vi "spill_param_tcp_server_v2.vi"(6 "error in":errorcluster, 8 "spill_id_Refnum":refnum<vi>, 9 "EOS_Refnum":refnum<vi>, 10 "BOS_Refnum":refnum<vi>, 11 "port":i16=9999) -> (4 "error out":errorcluster)   [LabVIEW 2019]
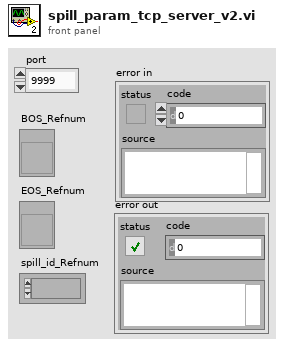
[diagram p1: front panel]
types:
  T1 = enum16{"Standard", "Buffered", "CRLF", "Immediate"}
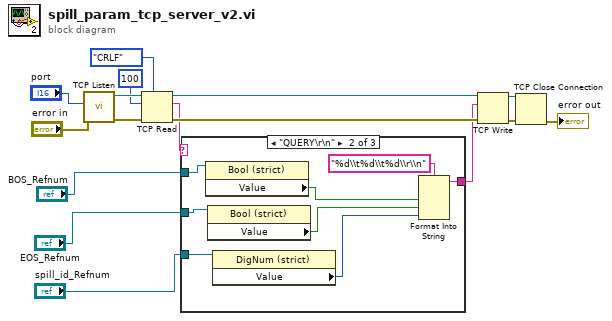
[diagram p0: block diagram]
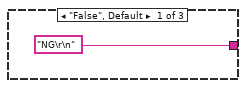
[diagram p2: hidden frame]
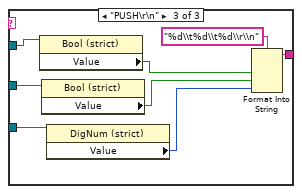
[diagram p3: hidden frame]
diagram:
  n1 = call <vilib>:"TCP Listen.vi"("error in (no error)"="error in", "port"="port") -> ("error out"=w16:errorcluster, "connection ID"=w15:refnum<k5>)  [unwired: 5 in, 3 out]
  n2 = TCP Read(connection ID=w15, bytes to read=100, error in (no error)=w16, 7:T1."CRLF" ("mode (standard)")) -> (connection ID out=w13:refnum<k5>, data out=w6:string, error out=w14:errorcluster)  [unwired: 1 in]
  n3 = case shown="\"QUERY\\r\\n\"" w6 {
    tunnel: ["NG\r\n" w24 w32] -> w9
    tunnel: "BOS_Refnum" -> [_ w23 w31]
    tunnel: "EOS_Refnum" -> [_ w21 w30]
    tunnel: "spill_id_Refnum" -> [_ w19 w29]
    frame "False", Default {
    }
    frame "QUERY\r\n" {
      n4 = property on="Property Node" class="Bool (strict)"(reference=w23) -> ("Value"=w22:bool)  [unwired: 1 in, 2 out]
      n5 = property on="Property Node" class="Bool (strict)"(reference=w21) -> ("Value"=w20:bool)  [unwired: 1 in, 2 out]
      n6 = property on="Property Node" class="DigNum (strict)"(reference=w19) -> ("Value"=w18:i32)  [unwired: 1 in, 2 out]
      n7 = Format Into String(format string="%d\\t%d\\t%d\\r\\n", w22, w20, w18) -> (resulting string=w24:string)  [unwired: 2 in, 1 out]
    }
    frame "PUSH\r\n" {
      n8 = property on="Property Node" class="Bool (strict)"(reference=w31) -> ("Value"=w28:bool)  [unwired: 1 in, 2 out]
      n9 = property on="Property Node" class="Bool (strict)"(reference=w30) -> ("Value"=w27:bool)  [unwired: 1 in, 2 out]
      n10 = property on="Property Node" class="DigNum (strict)"(reference=w29) -> ("Value"=w26:i32)  [unwired: 1 in, 2 out]
      n11 = Format Into String(format string="%d\\t%d\\t%d\\r\\n", w28, w27, w26) -> (resulting string=w32:string)  [unwired: 2 in, 1 out]
    }
  }
  n12 = TCP Write(connection ID=w13, data in=w9, error in (no error)=w14) -> (connection ID out=w11:refnum<k5>, error out=w12:errorcluster)  [unwired: 1 in, 1 out]
  n13 = TCP Close Connection(connection ID=w11, error in (no error)=w12) -> (error out=→"error out":errorcluster)  [unwired: 1 in, 1 out]
